vi "STOPPED FUNCTION - Buffered_INCREMENT TIME.vi"(8 "Error In Cluster":T3={"Unhandled Error"=FALSE, "Error"={"status"=FALSE, "code"=0, "source"=""}, "Message Type"=enum."Code", "Number of Values"=0, "Msg Value Type"=[], "Msg Ints"=[], "Msg Real Values"=[], "Msg String Values"=[], "Severity (Emergency)"=enum."Emergency"} {"Msg Real Values" format="%.2f"}, 10 "Tags":T1[](array[typedef]), 11 "Source":refnum<class "Source.lvclass">) -> (0 "Error Out Cluster":T2={"Unhandled Error"=FALSE, "Error"={"status"=FALSE, "code"=0, "source"=""}, "Message Type"=enum."Code", "Number of Values"=0, "Msg Value Type"=[], "Msg Ints"=[], "Msg Real Values"=[], "Msg String Values"=[], "Severity (Emergency)"=enum."Emergency"} {"Msg Real Values" format="%.2f"})   [LabVIEW 2013, in "Customer.TestSLATE.Mnemonic.lvlib"]
uses:
  Customer.TestSLATE.Mnemonic.lvlib
  <vilib>/Test SLATE/CONTROLS/Error In Cluster.ctl
  <vilib>/Test SLATE/CONTROLS/Error Out Cluster.ctl
  <vilib>/Test SLATE/CLASSES/SOURCE/Source.lvclass
  <vilib>/Test SLATE/CVT/Tag Information.ctl
  <vilib>/Test SLATE/CLASSES/TAG/TS_Tag.lvclass
  <vilib>/Test SLATE/COMMON/Test Executive Commonl.vi
  <vilib>/Test SLATE/BUF_AI/Write AI Raw to Data Storage Init and Increment.vi
  <vilib>/Test SLATE/BUF_FI/Write FI Raw to Data Storage Init and Increment.vi
  <vilib>/Test SLATE/BUF_CA/Write CA Raw to Data Storage Init and Increment.vi
  <vilib>/Test SLATE/BUF_DI/Write DI Raw to Data Storage Init and Increment.vi
  <vilib>/Test SLATE/BUF_AO/Write AO Raw to Data Storage Init and Increment.vi
  <vilib>/Test SLATE/BUF_CH/Write CH Raw to Data Storage Init and Increment.vi
  <vilib>/Test SLATE/CVT_DO/DO Common Array.vi
  <vilib>/Test SLATE/BUF_DO/Write DO Raw to Data Storage Init and Increment.vi
  <vilib>/Test SLATE/Test SLATE.lvlib
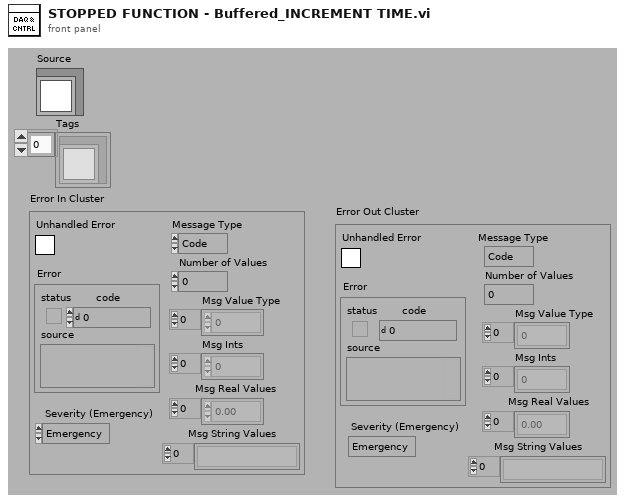
[diagram p1: front panel]
types:
  T1 = typedef "Test SLATE.lvlib/Tag Information.ctl" = refnum<class "TS_Tag.lvclass">
  T2 = typedef "Test SLATE.lvlib/Error Out Cluster.ctl" = cluster{"Unhandled Error":bool, "Error":errorcluster, "Message Type":enum8{"Code", "Text"}, "Number of Values":i8, "Msg Value Type":i32[], "Msg Ints":i32[], "Msg Real Values":sgl[], "Msg String Values":string[], "Severity (Emergency)":enum32{"Information", "Warning", "Emergency"}}
  T3 = typedef "Test SLATE.lvlib/Error In Cluster.ctl" = cluster{"Unhandled Error":bool, "Error":errorcluster, "Message Type":enum8{"Code", "Text"}, "Number of Values":i8, "Msg Value Type":i32[], "Msg Ints":i32[], "Msg Real Values":sgl[], "Msg String Values":string[], "Severity (Emergency)":enum32{"Information", "Warning", "Emergency"}}
  T4 = cluster{"Last Error":i32, "Error Active":bool, "AI Chan Status":i32[], "FI Chan Status":i32[], "CA Chan Status":i32[], "AO Chan Status":i32[], "DI Chan Status":i32[], "DO Chan Status":i32[], "CH Chan Status":i32[]}
  T5 = cluster{"AI Tag Offset":i32, "FI Tag Offset":i32, "DI Tag Offset":i32, "AO Tag Offset":i32, "DO Tag Offset":i32, "CA Tag Offset":i32, "CH Tag Offset":i32}
  T6 = cluster{"AI Tag Count":i16, "FI Tag Count":i16, "DI Tag Count":i16, "AO Tag Count":i16, "DO Tag Count":i16, "CA Tag Count":i16, "CH Tag Count":i16}
  T7 = typedef "Customer.TestSLATE.Mnemonic.lvlib/Source Status Information.ctl" = cluster{"Indexes":i32[], "Names":string[], "Bad Codes":bool[], "Low Ranges":sgl[], "High Ranges":sgl[]}
  T8 = enum16{"Started", "Stopped", "Initializing", "Acquiring", "Calibrating", "Diagnostics", "Inactive"}
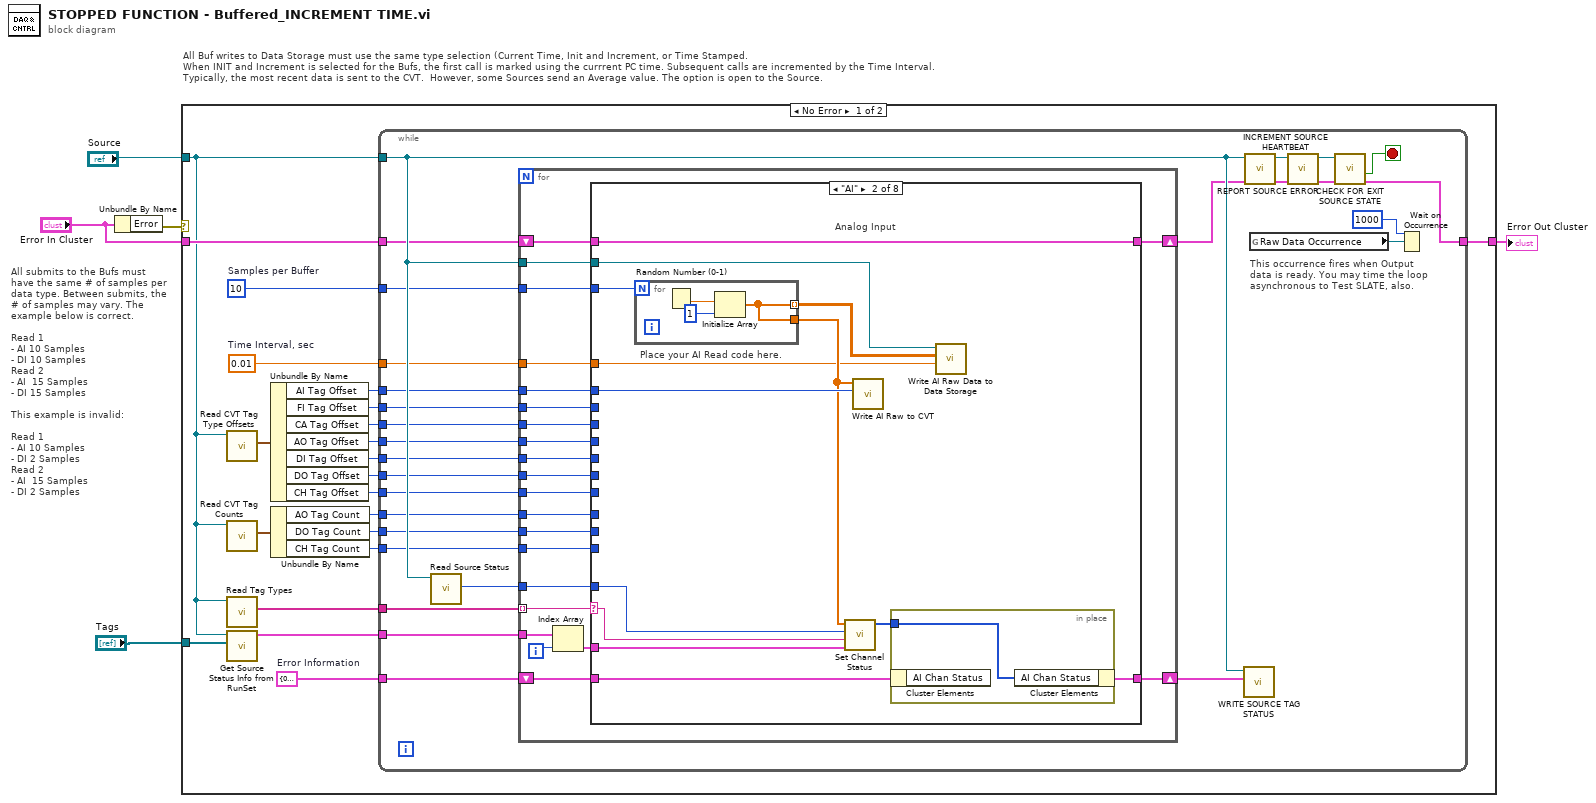
[diagram p0: block diagram]
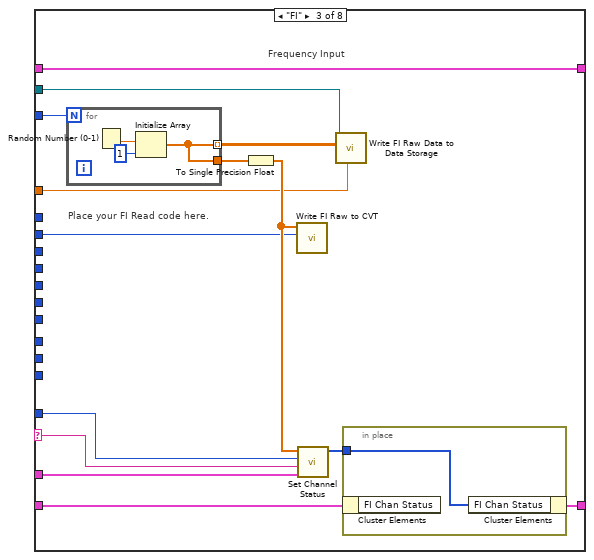
[diagram p3: hidden frame]
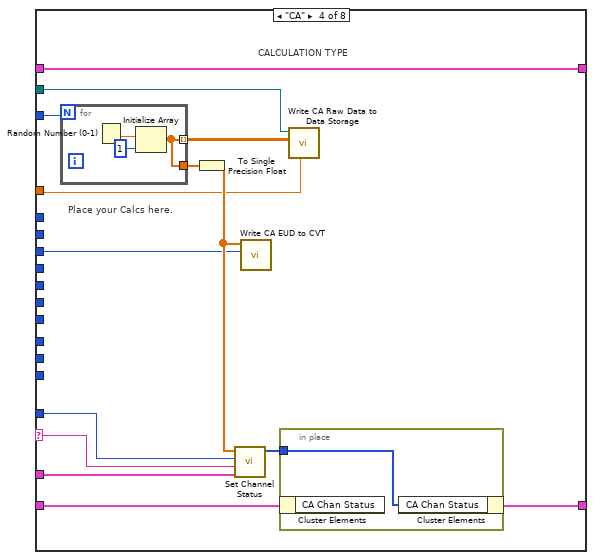
[diagram p4: hidden frame]
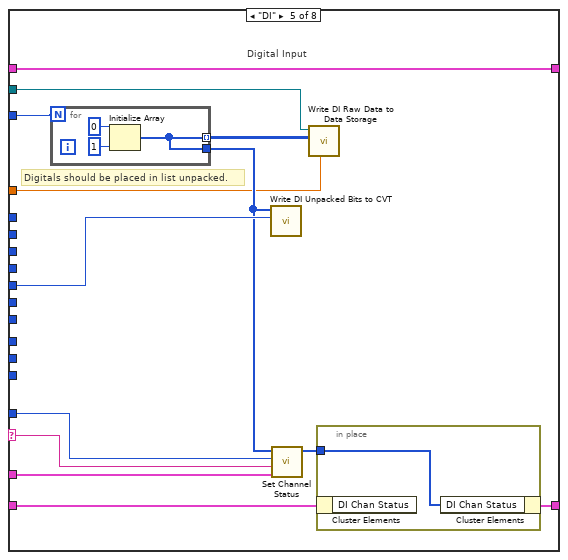
[diagram p5: hidden frame]
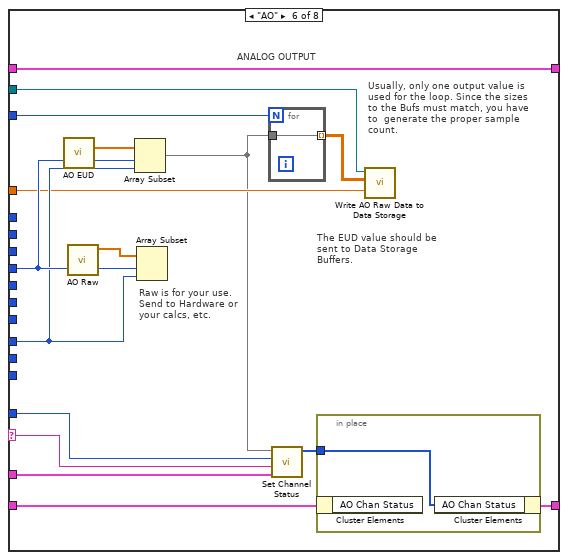
[diagram p6: hidden frame]
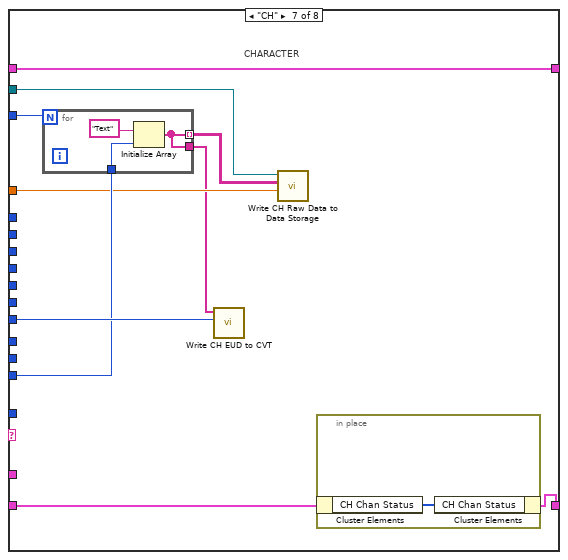
[diagram p7: hidden frame]
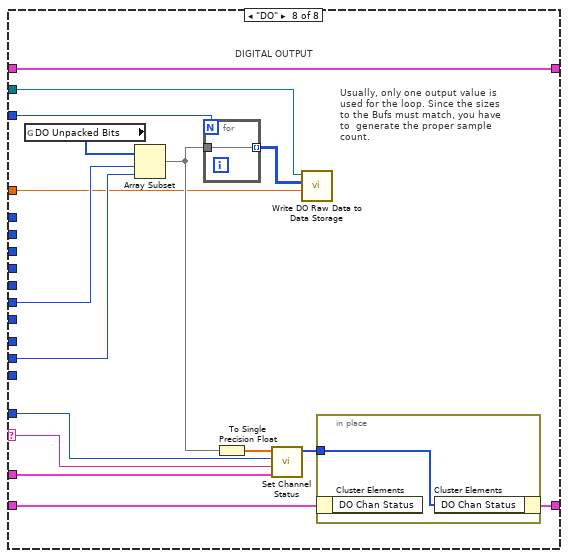
[diagram p8: hidden frame]
diagram:
  # "All Buf writes to Data Storage must use the same type selection (Current Time, Init and Increment, or Time Stamped.\nWhen INIT and Increment is selected for the Bufs, the first call is marked using the currrent PC time. Subsequent calls are incremented by the Time Interval.\nTypically, the most recent data is sent to the CVT.  However, some Sources send an Average value. The option is open to the Source."
  # "All submits to the Bufs must have the same # of samples per data type. Between submits, the # of samples may vary. The example below is correct.\n\nRead 1 \n- AI 10 Samples\n- DI 10 Samples\nRead 2 \n- AI  15 Samples\n- DI 15 Samples\n\nThis example is invalid:\n\nRead 1 \n- AI 10 Samples\n- DI 2 Samples\nRead 2 \n- AI  15 Samples\n- DI 2 Samples"
  n1 = Unbundle By Name("Error In Cluster") -> ("Error"=w5:errorcluster)
  n2 = case shown="No Error" w5 {
    tunnel: [w25 w199] -> w3
    tunnel: "Error In Cluster" -> [w26 w199]
    tunnel: "Source" -> [w9 _]
    tunnel: "Tags" -> [w22 _]
    frame No Error {
      w6 = 0.01  # Time Interval, sec
      w7 = 10  # Samples per Buffer
      w19 = T4 {"Last Error"=0, "Error Active"=FALSE, "AI Chan Status"=[], "FI Chan Status"=[], "CA Chan Status"=[], "AO Chan Status"=[], "DI Chan Status"=[], "DO Chan Status"=[], "CH Chan Status"=[]}  # Error Information
      n3 = call <vilib>:"Read CVT Tag Type Offsets.vi"("Source in"=w9) -> ("CVT Tag Offsets"=w24:T5)  [unwired: 9 in, 1 out]
      n4 = call <vilib>:"Read CVT Tag Counts.vi"("Source in"=w9) -> ("Tag Counts"=w12:T6)  [unwired: 9 in, 1 out]
      n5 = call <vilib>:"Read Tag Types.vi"("Source in"=w9) -> ("Tag Types"=w20:string[])  [unwired: 9 in, 1 out]
      n6 = call "Get Source Status Info from RunSet.vi"("Tags"=w22, "Source"=w9) -> ("Tag Status Info"=w21:T7[])  [unwired: 9 in]
      n7 = Unbundle By Name(w24) -> ("AI Tag Offset"=w23:i32, "FI Tag Offset"=w18:i32, "CA Tag Offset"=w17:i32, "AO Tag Offset"=w16:i32, "DI Tag Offset"=w15:i32, "DO Tag Offset"=w14:i32, "CH Tag Offset"=w13:i32)
      n8 = Unbundle By Name(w12) -> ("AO Tag Count"=w11:i16, "DO Tag Count"=w10:i16, "CH Tag Count"=w8:i16)
      n9 = while {
        tunnel: w26 -> [w38]
        tunnel: [w32] -> w25
        tunnel: w23 -> [w50]
        tunnel: w9 -> [w54]
        tunnel: w21 -> [w48]
        tunnel: w20 -> [w49]
        tunnel: w19 -> [w47]
        tunnel: w18 -> [w46]
        tunnel: w17 -> [w45]
        tunnel: w16 -> [w44]
        tunnel: w15 -> [w43]
        tunnel: w14 -> [w42]
        tunnel: w13 -> [w41]
        tunnel: w11 -> [w40]
        tunnel: w10 -> [w39]
        tunnel: w8 -> [w29]
        tunnel: w7 -> [w28]
        tunnel: w6 -> [w27]
        stop <- w53 stop-if-true
        # "This occurrence fires when Output\ndata is ready. You may time the loop asynchronous to Test SLATE, also."
        n10 = call <vilib>:"Read Source Status.vi"("Source in"=w54) -> ("Source Status"=w37:T8)  [unwired: 9 in, 1 out]
        n11 = for {
          tunnel: w50 -> [w67]
          tunnel: w54 -> [w76]
          tunnel: w49 -> [w75] mode=indexing
          tunnel: w48 -> [w74]
          shift-right: [w69] -> w30
          shift-left: w47 -> [w71]
          tunnel: w37 -> [w70]
          tunnel: w46 -> [w68]
          tunnel: w45 -> [w66]
          tunnel: w44 -> [w65]
          tunnel: w43 -> [w64]
          tunnel: w42 -> [w63]
          tunnel: w41 -> [w62]
          tunnel: w40 -> [w61]
          tunnel: w39 -> [w60]
          shift-right: [w58] -> w36
          shift-left: w38 -> [w59]
          tunnel: w29 -> [w57]
          tunnel: w28 -> [w56]
          tunnel: w27 -> [w55]
          i -> [w73]
          n12 = Index Array(array=w74, index=w73) -> (element=w72:T7)
          n13 = case shown="\"AI\"" w75 {
            selector: w75 -> [_ w88 w106 w124 w142 w162 _ w193]
            tunnel: w67 -> [_ w91 _ _ _ _ _ _]
            tunnel: w76 -> [_ w90 w109 w127 w144 w164 w176 w196]
            tunnel: w72 -> [_ w89 w107 w125 w143 w163 _ w194]
            tunnel: w71 -> [w78 w85 w103 w121 w139 w159 w175 w190]
            tunnel: w70 -> [_ w86 w104 w122 w140 w160 _ w191]
            tunnel: [w78 w84 w102 w120 w138 w158 w174 w189] -> w69
            tunnel: w68 -> [_ _ w101 _ _ _ _ _]
            tunnel: w66 -> [_ _ _ w119 _ _ _ _]
            tunnel: w65 -> [_ _ _ _ _ w154 _ _]
            tunnel: w64 -> [_ _ _ _ w137 _ _ _]
            tunnel: w63 -> [_ _ _ _ _ _ _ w187]
            tunnel: w62 -> [_ _ _ _ _ _ w172 _]
            tunnel: w61 -> [_ _ _ _ _ w153 _ _]
            tunnel: w60 -> [_ _ _ _ _ _ _ w186]
            tunnel: [w77 w83 w100 w118 w136 w157 w173 w185] -> w58
            tunnel: w59 -> [w77 w83 w100 w118 w136 w157 w173 w185]
            tunnel: w57 -> [_ _ _ _ _ _ w171 _]
            tunnel: w56 -> [_ w82 w99 w117 w135 w152 w170 w181]
            tunnel: w55 -> [_ w79 w97 w114 w132 w151 w169 w182]
            frame "", Default {
            }
            frame "AI" {
              # "Place your AI Read code here."
              # "Analog Input"
              n14 = for {
                N: w82 -> [_]
                tunnel: [w92] -> w80 mode=indexing
                tunnel: [w92] -> w81
                n15 = Random Number (0-1)() -> (number: 0 to 1=w94:dbl)
                n16 = Initialize Array(w94, 1 ("dimension size")) -> (w92:dbl[])
              }
              n17 = call "Set Channel Status.vi"("Status Info"=w89, "Data Type"=w88, "My System Status"=w86, "Real Data"=w81) -> ("Channel Statuses"=w87:u32[])  [unwired: 7 in]
              n18 = call <vilib>:"Write AI Raw to CVT.vi"("Start Type Index"=w91, "AI Raw"=w81) -> ()  [unwired: 10 in]
              n19 = in-place {
                in-place-border: w87 -> [w95]
                n20 = in-place-cluster #1(w85) -> ()  [unwired: 1 out]
                n21 = in-place-cluster #1("AI Chan Status"=w95) -> (w84:T4)
              }
              n22 = call-poly <vilib>:"Write AI Raw Data to Data Storage.vi"("Time Interval"=w79, "Analog Input Data"=w80, "Source"=w90) -> ()  [unwired: 9 in]
            }
            frame "FI" {
              # "Place your FI Read code here."
              # "Frequency Input"
              n23 = for {
                N: w99 -> [_]
                tunnel: [w110] -> w98 mode=indexing
                tunnel: [w110] -> w96
                n24 = Random Number (0-1)() -> (number: 0 to 1=w112:dbl)
                n25 = Initialize Array(w112, 1 ("dimension size")) -> (w110:dbl[])
              }
              n26 = To Single Precision Float(number=w96) -> (single precision float=w108:sgl[])
              n27 = call <vilib>:"Write FI Raw to CVT.vi"("Start Type Index"=w101, "FI Raw"=w108) -> ()  [unwired: 10 in]
              n28 = call "Set Channel Status.vi"("Status Info"=w107, "Data Type"=w106, "My System Status"=w104, "Real Data"=w108) -> ("Channel Statuses"=w105:u32[])  [unwired: 7 in]
              n29 = call-poly <vilib>:"Write FI Raw Data to Data Storage.vi"("Time Interval"=w97, "Frequency Input Data"=w98, "Source"=w109) -> ()  [unwired: 9 in]
              n30 = in-place {
                in-place-border: w105 -> [w113]
                n31 = in-place-cluster #2(w103) -> ()  [unwired: 1 out]
                n32 = in-place-cluster #2("FI Chan Status"=w113) -> (w102:T4)
              }
            }
            frame "CA" {
              # "Place your Calcs here."
              # "CALCULATION TYPE"
              n33 = for {
                N: w117 -> [_]
                tunnel: [w128] -> w116 mode=indexing
                tunnel: [w128] -> w115
                n34 = Random Number (0-1)() -> (number: 0 to 1=w130:dbl)
                n35 = Initialize Array(w130, 1 ("dimension size")) -> (w128:dbl[])
              }
              n36 = To Single Precision Float(number=w115) -> (single precision float=w126:sgl[])
              n37 = call "Set Channel Status.vi"("Status Info"=w125, "Data Type"=w124, "My System Status"=w122, "Real Data"=w126) -> ("Channel Statuses"=w123:u32[])  [unwired: 7 in]
              n38 = call <vilib>:"Write CA EUD to CVT.vi"("Start Type Index"=w119, "CA CAL EUD"=w126) -> ()  [unwired: 10 in]
              n39 = in-place {
                in-place-border: w123 -> [w131]
                n40 = in-place-cluster #3(w121) -> ()  [unwired: 1 out]
                n41 = in-place-cluster #3("CA Chan Status"=w131) -> (w120:T4)
              }
              n42 = call-poly <vilib>:"Write CA Raw Data to Data Storage.vi"("Time Interval"=w114, "Calculated Input Data"=w116, "Source"=w127) -> ()  [unwired: 9 in]
            }
            frame "DI" {
              # "Digitals should be placed in list unpacked."
              # "Digital Input"
              n43 = for {
                N: w135 -> [_]
                tunnel: [w145] -> w134 mode=indexing
                tunnel: [w145] -> w133
                n44 = Initialize Array(u32 0 ("element"), 1 ("dimension size")) -> (w145:u32[])
              }
              n45 = call <vilib>:"Write DI Unpacked Bits to CVT.vi"("Start Type Index"=w137, "DI EUD"=w133) -> ()  [unwired: 10 in]
              n46 = call "Set Channel Status.vi"("Status Info"=w143, "Data Type"=w142, "My System Status"=w140, "Real Data"=w133) -> ("Channel Statuses"=w141:u32[])  [unwired: 7 in]
              n47 = call-poly <vilib>:"Write DI Raw Data to Data Storage.vi"("Time Interval"=w132, "Digital Input Data"=w134, "Source"=w144) -> ()  [unwired: 9 in]
              n48 = in-place {
                in-place-border: w141 -> [w148]
                n49 = in-place-cluster #4(w139) -> ()  [unwired: 1 out]
                n50 = in-place-cluster #4("DI Chan Status"=w148) -> (w138:T4)
              }
            }
            frame "AO" {
              # "Usually, only one output value is used for the loop. Since the sizes to the Bufs must match, you have to  generate the proper sample count."
              # "The EUD value should be sent to Data Storage Buffers."
              # "Raw is for your use. Send to Hardware or your calcs, etc."
              # "ANALOG OUTPUT"
              n51 = call <vilib>:"AO EUD.vi"() -> ("AO EUD"=w156:sgl[])  [unwired: 3 in]
              n52 = call <vilib>:"AO Raw.vi"() -> ("AO Raw"=w155:sgl[])  [unwired: 11 in]
              n53 = Array Subset(array=w156, index=w154, length=w153) -> (w149:sgl[])
              n54 = Array Subset(array=w155, index=w154, length=w153) -> ()  [unwired: 1 out]
              n55 = for {
                N: w152 -> [_]
                tunnel: [w165] -> w150 mode=indexing
                tunnel: w149 -> [w165]
              }
              n56 = call "Set Channel Status.vi"("Status Info"=w163, "Data Type"=w162, "My System Status"=w160, "Real Data"=w149) -> ("Channel Statuses"=w161:u32[])  [unwired: 7 in]
              n57 = in-place {
                in-place-border: w161 -> [w166]
                n58 = in-place-cluster #5(w159) -> ()  [unwired: 1 out]
                n59 = in-place-cluster #5("AO Chan Status"=w166) -> (w158:T4)
              }
              n60 = call-poly <vilib>:"Write AO Raw Data to Data Storage.vi"("Time Interval"=w151, "Analog Output EUD"=w150, "Source"=w164) -> ()  [unwired: 9 in]
            }
            frame "CH" {
              # "CHARACTER"
              n61 = for {
                N: w170 -> [_]
                tunnel: [w177] -> w168 mode=indexing
                tunnel: w171 -> [w178]
                tunnel: [w177] -> w167
                n62 = Initialize Array("Text", w178) -> (w177:string[])
              }
              n63 = call <vilib>:"Write CH EUD to CVT.vi"("Start Type Index"=w172, "CH Text"=w167) -> ()  [unwired: 10 in]
              n64 = call-poly <vilib>:"Write CH Raw Data to Data Storage.vi"("Time Interval"=w169, "Character Data"=w168, "Source"=w176) -> ()  [unwired: 9 in]
              n65 = in-place {
                n66 = in-place-cluster #6(w175) -> ("CH Chan Status"=w180:i32[])
                n67 = in-place-cluster #6("CH Chan Status"=w180) -> (w174:T4)
              }
            }
            frame "DO" {
              # "Usually, only one output value is used for the loop. Since the sizes to the Bufs must match, you have to  generate the proper sample count."
              # "DIGITAL OUTPUT"
              n68 = global read "DO Common Array.vi" "DO Unpacked Bits"() -> (w188:i16[])
              n69 = Array Subset(array=w188, index=w187, length=w186) -> (w184:i16[])
              n70 = for {
                N: w181 -> [_]
                tunnel: [w197] -> w183 mode=indexing
                tunnel: w184 -> [w197]
              }
              n71 = To Single Precision Float(number=w184) -> (single precision float=w195:sgl[])
              n72 = call "Set Channel Status.vi"("Status Info"=w194, "Data Type"=w193, "My System Status"=w191, "Real Data"=w195) -> ("Channel Statuses"=w192:u32[])  [unwired: 7 in]
              n73 = call-poly <vilib>:"Write DO Raw Data to Data Storage.vi"("Time Interval"=w182, "Digital Output Data"=w183, "Source"=w196) -> ()  [unwired: 9 in]
              n74 = in-place {
                in-place-border: w192 -> [w198]
                n75 = in-place-cluster #7(w190) -> ()  [unwired: 1 out]
                n76 = in-place-cluster #7("DO Chan Status"=w198) -> (w189:T4)
              }
            }
          }
        }
        n77 = call <vilib>:"WRITE SOURCE TAG STATUS.vi"("Error Information"=w30, "Source"=w54) -> ()  [unwired: 8 in, 2 out]
        n78 = call <vilib>:"INCREMENT SOURCE HEARTBEAT.vi"("Error In Cluster"=w36, "Source"=w54) -> ("Error Out Cluster"=w34:T2, "Source out"=w35:refnum<class "Source.lvclass">)  [unwired: 8 in]
        n79 = global read "Test Executive Commonl.vi" "Raw Data Occurrence"() -> (w52:refnum<k4>)
        n80 = call <vilib>:"REPORT SOURCE ERROR.vi"("Error In Cluster"=w34, "Source"=w35) -> ("Error Out Cluster"=w33:T2, "Source Out"=w31:refnum<class "Source.lvclass">)  [unwired: 8 in]
        n81 = call <vilib>:"CHECK FOR EXIT SOURCE STATE.vi"("Error In Cluster"=w33, "Source"=w31) -> ("Error Out Cluster"=w32:T2, "Exit Source State"=w53:bool)  [unwired: 7 in, 1 out]
        n82 = Wait on Occurrence(2:w52, 3:1000 ("ms timeout (-1)")) -> ()  [unwired: 1 in, 1 out]
      }
    }
    frame Error {
    }
  }
  "Error Out Cluster" <- w3
